vi "Histogram.vi"(0 "Image In":T1, 7 "error in":errorcluster) -> (20 "Image Out":T1, 27 "error out":errorcluster)   [LabVIEW 2009]
uses:
  <vilib>/vision/Image Controls.llb/IMAQ Image.ctl
panel:
  out "Histogram Graph":u32[][](graph)
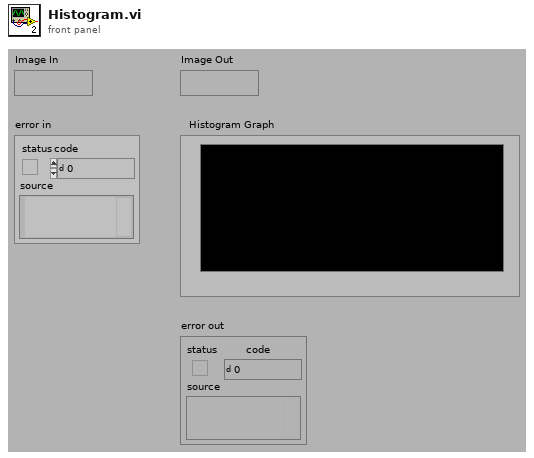
[diagram p1: front panel]
types:
  T1 = typedef "IMAQ Image.ctl" = refnum<image>
  T2 = cluster{"Global Rectangle":i32[], "Contours":cluster{"ID":enum32{"External", "Internal"}, "Type":u32, "Coordinates":i32[]}[]}
  T3 = cluster{"Minimal Value":sgl, "Maximal Value":sgl, "Mean Value":sgl, "Standard  Variation":sgl, "Area (pixels)":i32}
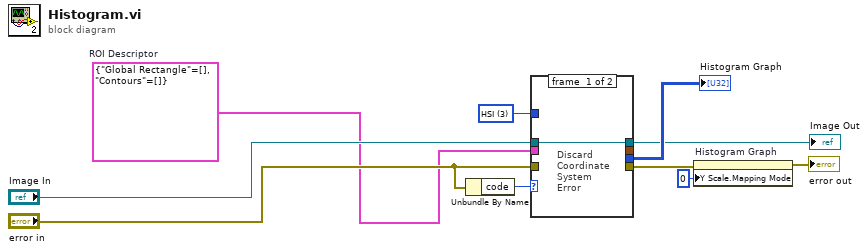
[diagram p0: block diagram]
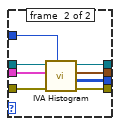
[diagram p2: hidden frame]
diagram:
  w6 = u16 3 items=["RGB", "HSL", "HSV", "HSI"] ("Color Mode")
  w4 = T2 {"Global Rectangle"=[], "Contours"=[]}  # ROI Descriptor
  n1 = Unbundle By Name("error in") -> ("code"=w1:i32)
  n2 = case shown="Default" w1 {
    tunnel: "error in" -> [_ w19]
    tunnel: "Image In" -> [w11 w18]
    tunnel: [_ w17] -> _
    tunnel: [_ w16] -> w7
    tunnel: w6 -> [_ w15]
    tunnel: [_ w14] -> w5
    tunnel: w4 -> [_ w13]
    tunnel: [w11 w12] -> w3
    frame #0 {
      # "Discard\nCoordinate\nSystem\nError"
    }
    frame #1 {
      n3 = call <vilib>:"IVA Histogram.vi"("Color Mode"=w15, "error in (no error)"=w19, "ROI Descriptor"=w13, "Image In"=w18) -> ("error out"=w16:errorcluster, "Histograms"=w14:u32[][], "Statistics"=w17:T3, "Image Out"=w12:T1)  [unwired: 4 out]
    }
  }
  "Image Out" <- w3
  "Histogram Graph" <- w5
  n4 = property on="Histogram Graph"(error in=w7, "Y Scale.Mapping Mode"=u8 0) -> (error out=→"error out":errorcluster)  [unwired: 1 in, 1 out]
